vi "I Doppler trigger signal using STFT PtByPt.vi"() -> ()   [LabVIEW 2022 SP3]
doc: "Performs real-time Joint Time Frequency Analysis (JTFA) using Point By Point STFT. The signal is simulated by a sine wave plus Gaussian noise."
uses:
  <vilib>/DAQmx/read.llb/DAQmx Read (Analog Wfm 1Chan 1Samp).vi
  <vilib>/DAQmx/miscellaneous.llb/DAQmx Fill In Error Info.vi
  <vilib>/measure/mamon.llb/Waveform Peak Detection for N Chan.vi
  <vilib>/ptbypt/NI_PtbyPt.lvlib
  <vilib>/measure/NI_MAPro.lvlib
  <resource>/objmgr/daqmx.rc
panel:
  in  "DAQmx Task Name":refnum<k21>
  out "Waveform Graph 4":dynamicdata(graph)
  out "Waveform Graph 3":dbl[](graph)
  out "Waveform Graph 2":dbl[](graph)
  out "locations time 1":dbl[](array[numeric])
  out "locations time 0":dbl[](array[numeric])
  out "Locations":cluster{"Locations":dbl[]}[](array[cluster]) {"Locations" format="%.2p"}
  out "Amplitudes":cluster{"Amplitudes":dbl[]}[](array[cluster]) {"Amplitudes" format="%.2p"}
  out "# peaks found":i32[](array[numeric])
  out "Waveform Graph":dbl[][](graph)
  out "Array 3":dbl[][](array[numeric])
  out "DT":dbl
  out "dt":dbl
  out "Number of cols (freq)":dbl
  out "Number of rows (time)":dbl
  out "Array 2":i32[](array[numeric])
  in  "time increment":i32=200
  out "Moving STFT":dbl[][](graph)
  in  "window length":i32=100 format="%0.0f"
  in  "stop":bool
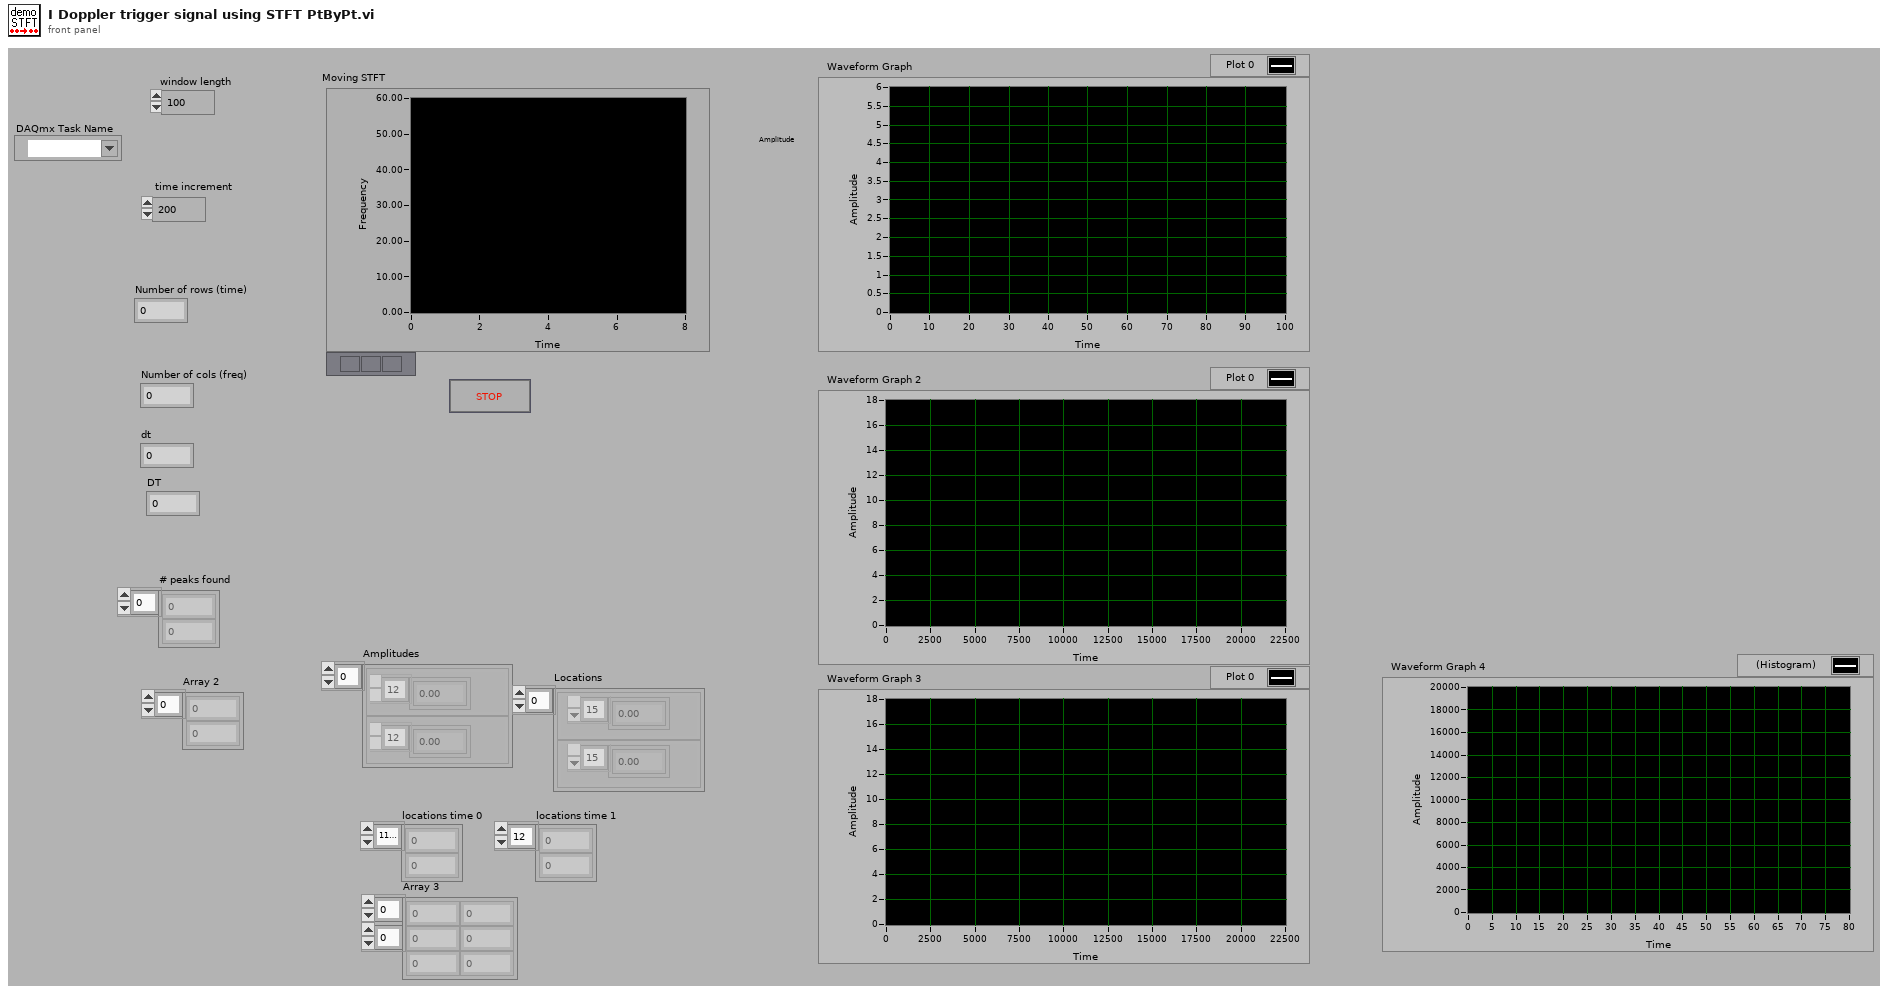
[diagram p1: front panel]
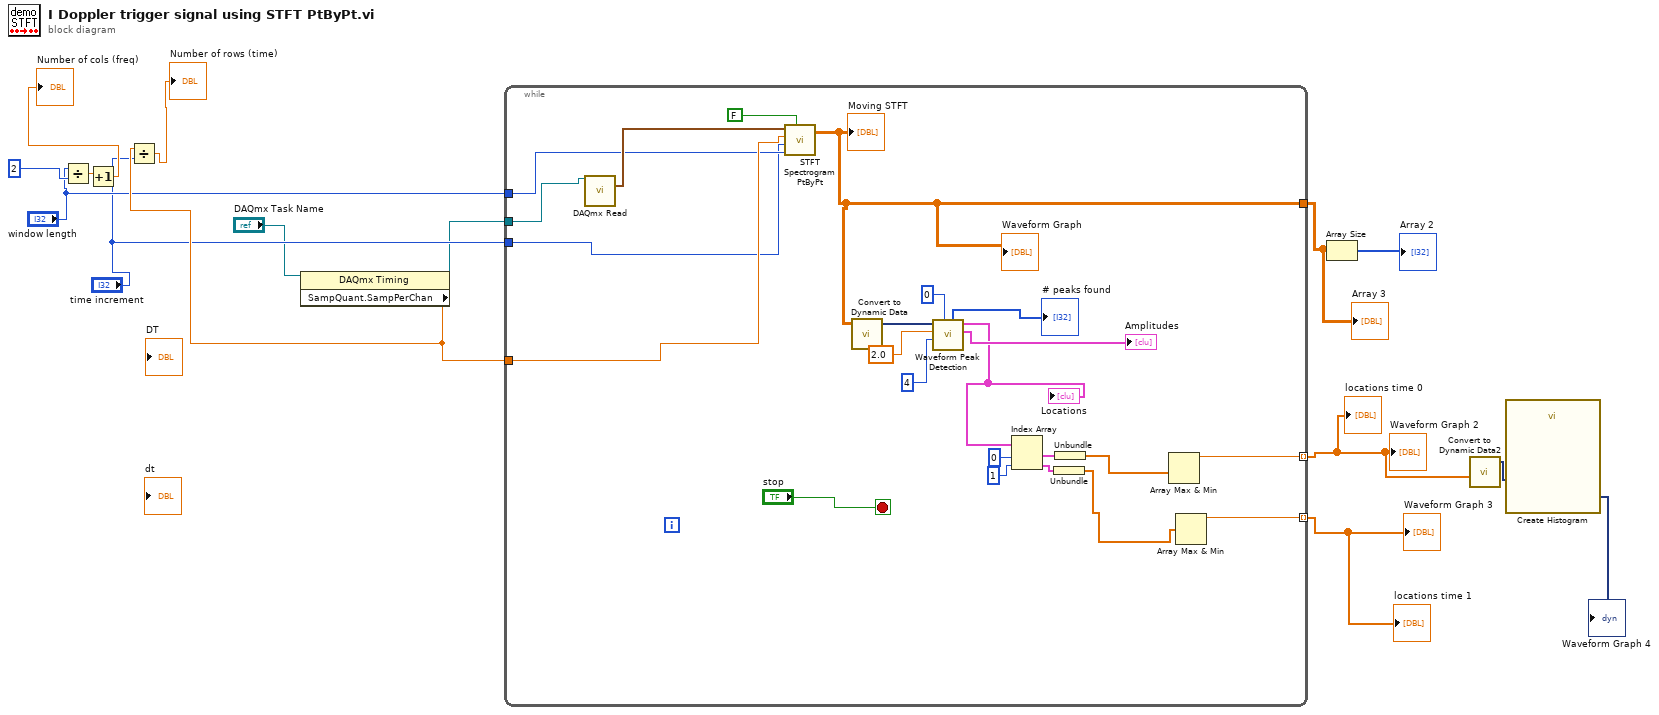
[diagram p0: block diagram]
diagram:
  n1 = Divide(x="window length", y=u32 2 ("milliseconds to wait")) -> (x/y=w14:dbl)
  n2 = Increment(x=w14) -> (x+1=→"Number of cols (freq)":dbl)
  n3 = property class="DAQmx Timing"(reference="DAQmx Task Name") -> (reference out=w1:refnum<k21>, "SampQuant.SampPerChan"=w5:dbl)  [unwired: 1 in, 1 out]
  n4 = Divide(x=w5, y="time increment") -> (x/y=→"Number of rows (time)":dbl)
  n5 = while {
    tunnel: [w16] -> w10
    tunnel: [w24] -> w8 mode=indexing
    tunnel: [w23] -> w9 mode=indexing
    tunnel: w1 -> [w22]
    tunnel: w5 -> [w19]
    tunnel: "window length" -> [w18]
    tunnel: "time increment" -> [w17]
    stop <- "stop" stop-if-true
    n6 = call-poly <vilib>:"DAQmx Read.vi"("task/channels in"=w22) -> ("data"=w21:waveform(dbl))  [unwired: 1 in, 13 out]
    n7 = call <vilib>:"STFT Spectrogram PtByPt.vi"("initialize"=FALSE, "window length"=w18, "time increment"=w17, "sample length"=w19, "x"=w21) -> ("STFT Spectrogram {X}"=w16:dbl[][])  [unwired: 1 in, 1 out]
    "Moving STFT" <- w16
    "Waveform Graph" <- w16
    n8 = call "Convert to Dynamic Data"("2D Array"=w16) -> ("Dynamic Data Type"=w37:dynamicdata)  [unwired: 3 out]
    n9 = call-poly <vilib>:"Waveform Peak Detection.vi"("peaks/valleys"=u32 0 ("milliseconds to wait"), "width"=u32 4 ("milliseconds to wait"), "threshold"=2.0 ("Y Scale.Range:Minimum"), "Signals In"=w37) -> ("Amplitudes"=→"Amplitudes":cluster{"Amplitudes":dbl[]}[], "Locations"=w31:cluster{"Locations":dbl[]}[], "# found"=→"# peaks found":i32[])  [unwired: 3 in, 2 out]
    "Locations" <- w31
    n10 = Index Array(array=w31, index #1=u32 0 ("milliseconds to wait"), index #2=u32 1 ("milliseconds to wait")) -> (element #1=w29:cluster{"Locations":dbl[]}, element #2=w27:cluster{"Locations":dbl[]})
    n11 = Unbundle(w27) -> ("Locations"=w25:dbl[])
    n12 = Unbundle(w29) -> ("Locations"=w26:dbl[])
    n13 = Array Max & Min(array=w26) -> (max value=w24:dbl)  [unwired: 3 out]
    n14 = Array Max & Min(array=w25) -> (max value=w23:dbl)  [unwired: 3 out]
  }
  "Array 3" <- w10
  "Waveform Graph 2" <- w8
  "Waveform Graph 3" <- w9
  "locations time 0" <- w8
  "locations time 1" <- w9
  n15 = Array Size(array=w10) -> (size(s)=→"Array 2":i32[])
  n16 = call "Convert to Dynamic Data2"("Array"=w8) -> ("Dynamic Data Type"=w7:dynamicdata)  [unwired: 3 out]
  n17 = call "Create Histogram"("Signal"=w7) -> ("Histogram"=→"Waveform Graph 4":dynamicdata)  [unwired: 3 in, 7 out]
